vi "test_save_1.vi"() -> ()   [LabVIEW 2016]
panel:
  out "text":string
  in  "Numeric":dbl
  in  "stop":bool
  out "String":string
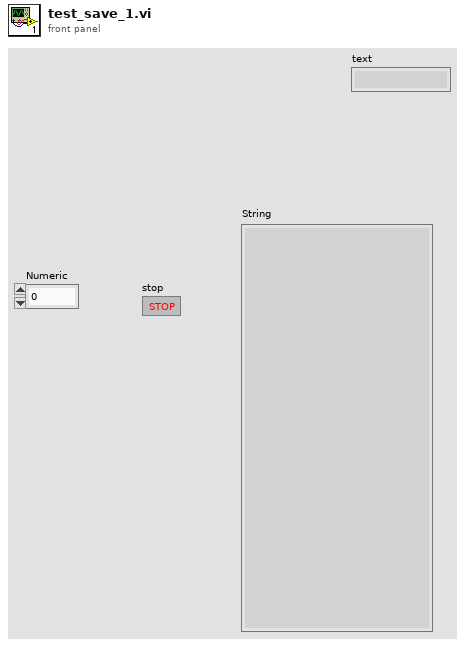
[diagram p1: front panel]
types:
  T1 = enum16{"open", "replace", "create", "open or create", "replace or create", "replace or create with confirmation"}
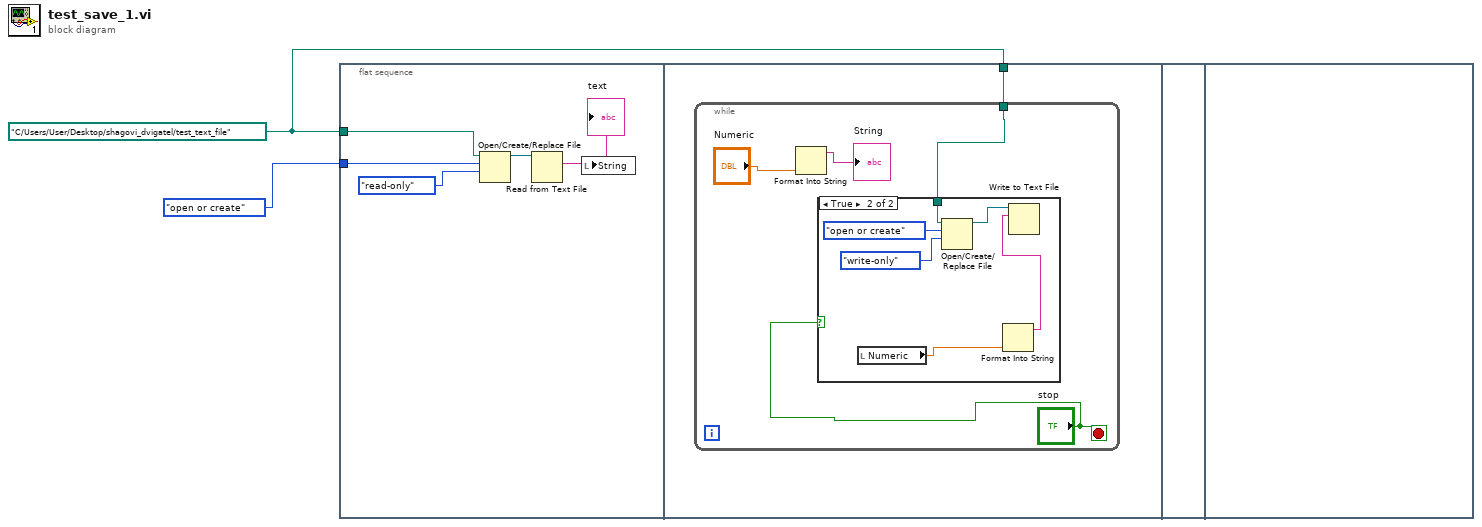
[diagram p0: block diagram]
diagram:
  w1 = path "C:/Users/User/Desktop/shagovi_dvigatel/test_text_file"
  n1 = flat-sequence {
    tunnel: T1."open or create" ("operation (0:open)") -> [w6]
    tunnel: w1 -> [w5]
    tunnel: w1 -> [w8]
    frame #0 {
      n2 = Open/Create/Replace File(file path (use dialog)=w5, operation (0:open)=w6, access (0:read/write)=enum16{"read/write", "read-only", "write-only"}."read-only") -> (refnum out=w7:refnum<file>)  [unwired: 3 in, 2 out]
      n3 = Read from Text File(file (use dialog)=w7) -> (text=w4:string)  [unwired: 3 in, 3 out]
      "text" <- w4
      n4 = local write "String"(w4) -> ()
    }
    frame #1 {
      n5 = while {
        tunnel: w8 -> [w9]
        stop <- "stop" stop-if-true
        n6 = Format Into String("Numeric") -> (resulting string=→"String":string)  [unwired: 3 in, 1 out]
        n7 = case shown="True" "stop" {
          tunnel: w9 -> [_ w15]
          frame False {
          }
          frame True {
            n8 = local read "Numeric"() -> (w14:dbl)
            n9 = Open/Create/Replace File(file path (use dialog)=w15, operation (0:open)=T1."open or create", access (0:read/write)=enum16{"read/write", "read-only", "write-only"}."write-only") -> (refnum out=w16:refnum<file>)  [unwired: 3 in, 2 out]
            n10 = Format Into String(w14) -> (resulting string=w13:string)  [unwired: 3 in, 1 out]
            n11 = Write to Text File(file (use dialog)=w16, text=w13) -> ()  [unwired: 2 in, 3 out]
          }
        }
      }
    }
    frame #2 {
    }
    frame #3 {
    }
  }
